vi "zero actuator.vi"(8 "error in":errorcluster, 11 "actuator in":T1={"Actuator COM"="COM14", "Actuator type"=enum."Scientifica"}) -> (0 "error out":errorcluster, 3 "actuator out":T1={"Actuator COM"="COM14", "Actuator type"=enum."Scientifica"})   [LabVIEW 2015]
uses:
  pipette cleaning/pressure box/cleaning_soft/controls/scientifica_commands.ctl
  pipette cleaning/pressure box/cleaning_soft/controls/actuator_type.ctl
  pipette cleaning/pressure box/cleaning_soft/controls/actuator_cluster.ctl
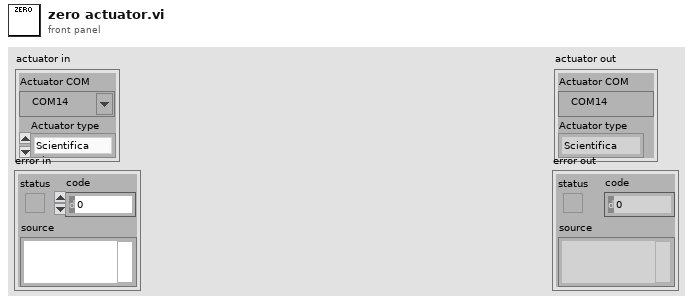
[diagram p1: front panel]
types:
  T1 = typedef "actuator_cluster.ctl" = cluster{"Actuator COM":refnum<visa-resource-name>, "Actuator type":T2}
  T2 = typedef "actuator_type.ctl" = enum16{"Scientifica", "Sutter", "Demo", "Off"}
  T3 = typedef "scientifica_commands.ctl" = enum16{"ANGLE", "INSET", "FIRST", "ZERO", "Pz", "P", "absz", "ACC", "TOP", "STOP", "rel", "relz", "abs", "IN", "vj", "APROACH", "OBJS", "OBJU", "OUT", "OBJ", "OBJL", "SET", "OBJD", "STEP", "SETSTEP", "S", "UUX", "UUY", "UUZ"}
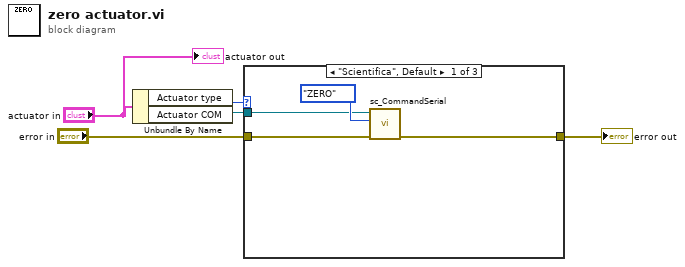
[diagram p0: block diagram]
diagram:
  n1 = Unbundle By Name("actuator in") -> ("Actuator type"=w3:T2, "Actuator COM"=w2:refnum<visa-resource-name>)
  n2 = case shown="\"Scientifica\", Default" w3 {
    tunnel: "error in" -> [w8 w10 w11]
    tunnel: w2 -> [w7 _ _]
    tunnel: [w6 w10 w11] -> w1
    frame "Scientifica", Default {
      n3 = call "sc_CommandSerial.vi"("error in (no error)"=w8, "Scientifica commands"=scientifica_commands."ZERO", "VISA handle"=w7) -> ("error out"=w6:errorcluster)  [unwired: 5 in, 3 out]
    }
    frame "Sutter" {
    }
    frame "Demo" {
    }
  }
  "error out" <- w1
  "actuator out" <- "actuator in"
